vi "Created Aliases.vi"(11 "jettl in":refnum<class "jettl.lvclass">) -> (2 "Created Aliases":T1)   [LabVIEW 2021, in "jettl.lvlib" / "jettl.lvclass"]
uses:
  jettl.lvclass
  Created Aliases.ctl
  jettl.lvlib
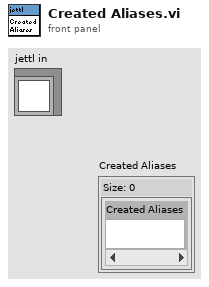
[diagram p1: front panel]
types:
  T1 = typedef "jettl.lvlib/Created Aliases.ctl" = set{string}
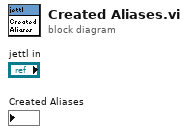
[diagram p0: block diagram]
diagram:
